vi "Force Close Log File Instance.vi"(8 "error in (no error)":errorcluster, 11 "Segmented Log in":refnum<class "Segmented Log.lvclass">) -> (0 "error out":errorcluster, 2 "Log Active":bool, 3 "Segmented Log out":refnum<class "Segmented Log.lvclass">)   [LabVIEW 2015, in "Segmented Log.lvclass"]
doc: "Closes the current log file instance if one is open, regardless of the specified segmenting limits."
uses:
  Segmented Log.lvclass
  Segmented Log.lvclass/Segmented Log.ctl
  Log Files/Log File/Log File.lvclass/Log File.ctl
  Log Files/TDMS Log File/TDMS Log File.lvclass/TDMS Log File.ctl
  Log Files/Text Log File/Text Log File.lvclass/Text Log File.ctl
  Log Files/Log File/Close Log File.vi
  Make File Read-Only.vi
  On Segmented Log Complete.vi
  On File Close.vi
  Log Files/TDMS Log File/Close TDMS Log File.vi
  Log Files/Text Log File/Close Text Log File.vi
  Log Files/Text Log File/Text Log File.lvclass
  Log Files/TDMS Log File/TDMS Log File.lvclass
  Log Files/Log File/Log File.lvclass
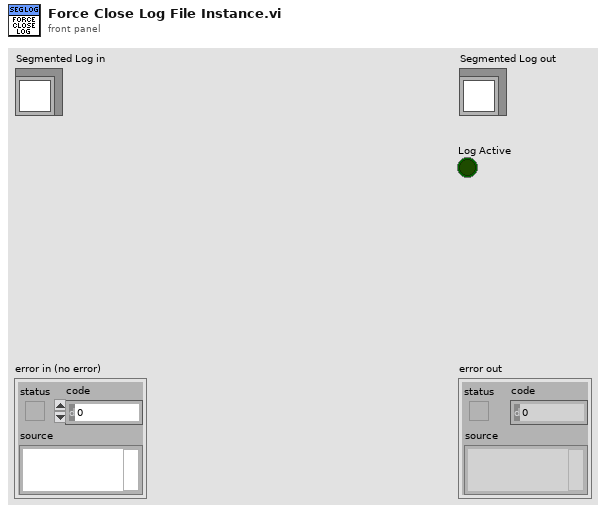
[diagram p1: front panel]
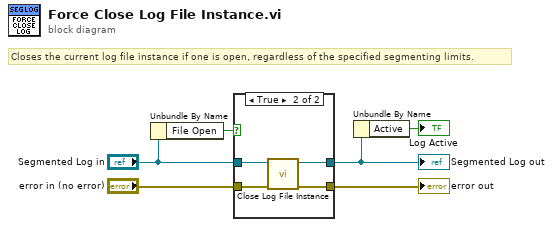
[diagram p0: block diagram]
diagram:
  # "Closes the current log file instance if one is open, regardless of the specified segmenting limits."
  n1 = Unbundle By Name("Segmented Log in") -> ("File Open"=w4:bool)
  n2 = case shown="True" w4 {
    tunnel: "error in (no error)" -> [w7 w12]
    tunnel: [w7 w11] -> w5
    tunnel: "Segmented Log in" -> [w8 w10]
    tunnel: [w8 w9] -> w2
    frame False {
    }
    frame True {
      n3 = call "Close Log File Instance.vi"("error in (no error)"=w12, "Segmented Log in"=w10) -> ("error out"=w11:errorcluster, "Segmented Log out"=w9:refnum<class "Segmented Log.lvclass">)  [unwired: 8 in]
    }
  }
  "error out" <- w5
  "Segmented Log out" <- w2
  n4 = Unbundle By Name(w2) -> ("Active"=→"Log Active":bool)
